vi "Testbench for Servo.vi"() -> ()   [LabVIEW 2011]
uses:
  <vilib>/FPGAPlugInAG/cRIO-9113/niLvFpga_Open_cRIO-9113.vi
  <vilib>/FPGAPlugInAG/cRIO-9113/niLvFpga_Close_cRIO-9113.vi
  <vilib>/rvi/interface/nirviOpenFPGA/nirviOpenFPGA.xnode
  FPGA Bitfiles/SailBot_FPGATarget_ReadFromFIFOPort_B155A09E.lvbitx
  1A-FPGA/1A Code/ReadFromFIFOPort4.vi
  <vilib>/rvi/interface/nirviCloseFPGA/nirviCloseFPGA.xnode
panel:
  in  "y":i32
  in  "y 2":dbl
  in  "stop":bool
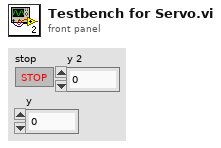
[diagram p1: front panel]
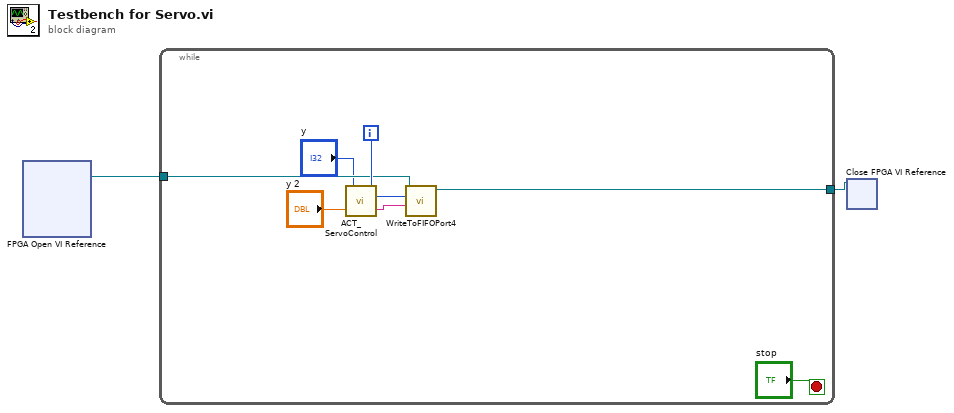
[diagram p0: block diagram]
diagram:
  n1 = xnode "FPGA Open VI Reference"() -> ("FPGA VI Reference Out"=w2:refnum<k20>)  [unwired: 2 in, 1 out]
  n2 = while {
    tunnel: w2 -> [w5]
    tunnel: [w4] -> w1
    i -> [w6]
    stop <- "stop" stop-if-true
    n3 = call "ACT_ServoControl.vi"("y 2"="y 2", "y"="y") -> ("String"=w7:string)  [unwired: 1 in]
    n4 = call "WriteToFIFOPort4.vi"("String"=w7, "loop#"=w6, "FPGA VI Reference Out"=w5) -> ("FPGA VI Reference Out 2"=w4:refnum<k20>)  [unwired: 8 in]
  }
  n5 = xnode "Close FPGA VI Reference"("FPGA VI Reference In"=w1) -> ()  [unwired: 1 in, 1 out]
